vi "build installer exe.vi"() -> ()   [LabVIEW 2016]
uses:
  <vilib>/AppBuilder/AB_API_Simple/Build Specification Version.ctl
  <vilib>/AppBuilder/AB_API_Simple/Set Build Specification Version (path).vi
  <vilib>/AppBuilder/AB_API_Simple/Build (path).vi
  <userlib>/LevyLab/Build Support/PostBuildSupport/PostBuildSupport.lvclass
  <vilib>/AppBuilder/AB_API_Simple/NI_App_Builder_API.lvlib
  <vilib>/MakerHub/Toolbox/LMH-Toolbox.lvlib
panel:
  in  "Build":u16=14
  in  "Fix":u16=6
  in  "Minor":u16=1
  in  "Major":u16=2
  # "Retrieve and Visualize\nTransconductance State Machine"
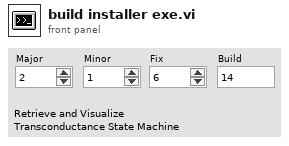
[diagram p1: front panel]
types:
  T1 = typedef "NI_App_Builder_API.lvlib/Build Specification Version.ctl" = cluster{"Major":u16, "Minor":u16, "Fix":u16, "Build":u16}
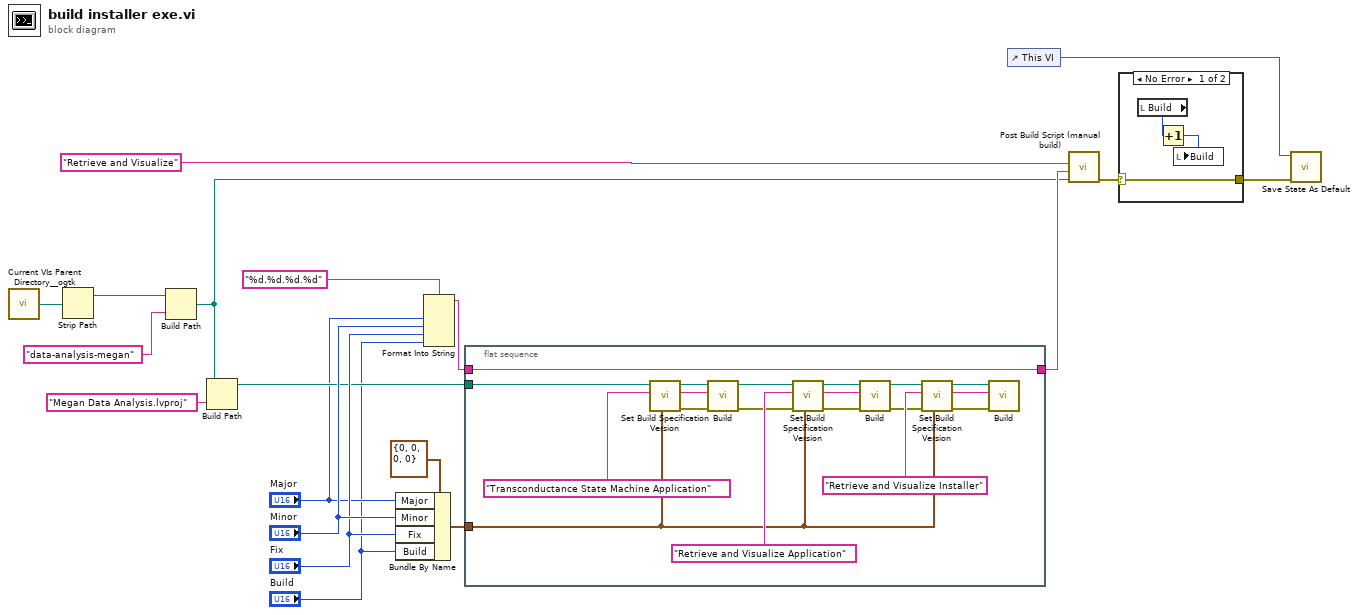
[diagram p0: block diagram]
diagram:
  n1 = call <userlib>:"Current VIs Parent Directory__ogtk.vi"() -> ("Parent Directory (+ Relative)"=w18:path)  [unwired: 5 in]
  n2 = Strip Path(path=w18) -> (stripped path=w17:path)  [unwired: 1 out]
  n3 = Build Path(base path=w17, name or relative path="data-analysis-megan") -> (appended path=w1:path)
  n4 = Build Path(base path=w1, name or relative path="Megan Data Analysis.lvproj") -> (appended path=w9:path)
  n5 = Bundle By Name(cluster=T1 {"Major"=0, "Minor"=0, "Fix"=0, "Build"=0} ("Build Specification Version"), "Major"="Major", "Minor"="Minor", "Fix"="Fix", "Build"="Build") -> (w13:T1)
  n6 = Format Into String(format string="%d.%d.%d.%d", "Major", "Minor", "Fix", "Build") -> (resulting string=w7:string)  [unwired: 2 in, 1 out]
  n7 = flat-sequence {
    tunnel: w13 -> [w25]
    tunnel: w9 -> [w27]
    tunnel: [w29] -> w6
    tunnel: w7 -> [w29]
    frame #0 {
      w26 = "Retrieve and Visualize Installer" ("Name of build specification")
      w30 = "Retrieve and Visualize Application" ("Name of build specification")
      w28 = "Transconductance State Machine Application" ("Name of build specification")
      n8 = call-poly <vilib>:"Set Build Specification Version.vi"("Build Specification Version"=w25, "Name of build specification"=w28, "Path to project"=w27) -> ("error out"=w24:errorcluster)  [unwired: 8 in]
      n9 = call-poly <vilib>:"Build.vi"("error in (no error)"=w24, "Name of build specification (if empty: build all)"=w28, "Path to project"=w27) -> ("error out"=w23:errorcluster)  [unwired: 7 in, 1 out]
      n10 = call-poly <vilib>:"Set Build Specification Version.vi"("Build Specification Version"=w25, "error in (no error)"=w23, "Name of build specification"=w30, "Path to project"=w27) -> ("error out"=w22:errorcluster)  [unwired: 7 in]
      n11 = call-poly <vilib>:"Build.vi"("error in (no error)"=w22, "Name of build specification (if empty: build all)"=w30, "Path to project"=w27) -> ("error out"=w20:errorcluster)  [unwired: 7 in, 1 out]
      n12 = call-poly <vilib>:"Set Build Specification Version.vi"("Build Specification Version"=w25, "error in (no error)"=w20, "Name of build specification"=w26, "Path to project"=w27) -> ("error out"=w21:errorcluster)  [unwired: 7 in]
      n13 = call-poly <vilib>:"Build.vi"("error in (no error)"=w21, "Name of build specification (if empty: build all)"=w26, "Path to project"=w27) -> ()  [unwired: 7 in, 2 out]
    }
  }
  n14 = control-ref of="This VI"() -> (w4:refnum<vi>)
  n15 = call <userlib>:"Post Build Script (manual build).vi"("Package Source Folder"=w1, "Package Version"=w6, "Product Name"="Retrieve and Visualize" ("Data Analysis")) -> ("error out"=w3:errorcluster)  [unwired: 8 in]
  n16 = case shown="No Error" w3 {
    selector: w3 -> [w33 w34]
    tunnel: [w33 w34] -> w2
    frame No Error {
      n17 = local read "Build"() -> (w32:u16)
      n18 = Increment(x=w32) -> (x+1=w31:u16)
      n19 = local write "Build"(w31) -> ()
    }
    frame Error {
    }
  }
  n20 = call <vilib>:"Save State As Default.vi"("Error In"=w2, "Target VI"=w4) -> ()  [unwired: 8 in, 2 out]
